vi "New.vi"(8 "Error In":errorcluster, 11 "Data":cluster{"Key":string, "Value":variant}[](array[cluster])) -> (0 "Error Out":errorcluster, 3 "Root":refnum<class "Root.lvclass">)   [LabVIEW 2018, in "Toolkit.lvlib" / "Nodes.lvlib" / "Root.lvclass"]
uses:
  Root.lvclass
  D:/Users/cfield/Code/Field R&D Services/Mustache/trunk/src/Toolkit/Nodes/NonTerminal/NonTerminal.lvclass
  NonTerminal/NonTerminal.lvclass/NonTerminal.ctl
  NonTerminal/NonTerminal.lvclass
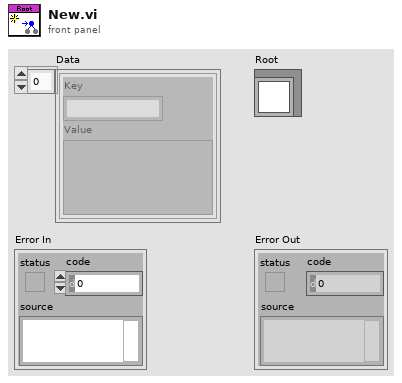
[diagram p1: front panel]
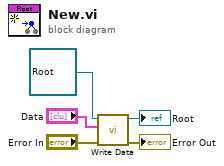
[diagram p0: block diagram]
diagram:
  n1 = call "Write Data.vi"("Error In"="Error In", "Data"="Data", "Non-Terminal In"=refnum<class "Root.lvclass"> refnum ("Toolkit.lvlib:Nodes.lvlib:Root.lvclass")) -> ("Error Out"=→"Error Out":errorcluster, "Non-Terminal Out"=→"Root":refnum<class "Root.lvclass">)  [unwired: 7 in]
